vi "获取公式.vi"(10 "量程选择":enum16{"L", "H", "AUTO"}(ring)) -> (2 "方程系数2":cluster{"X^2":dbl, "K":dbl, "b":dbl} {"X^2" format="%#.6g"; "b" format="%#.6g"; "K" format="%#.6g"}, 3 "方程系数":cluster{"X^2":dbl, "K":dbl, "b":dbl} {"X^2" format="%#.6g"; "b" format="%#.6g"; "K" format="%#.6g"})   [LabVIEW 2016, in "斯坦道CODMn.lvlib"]
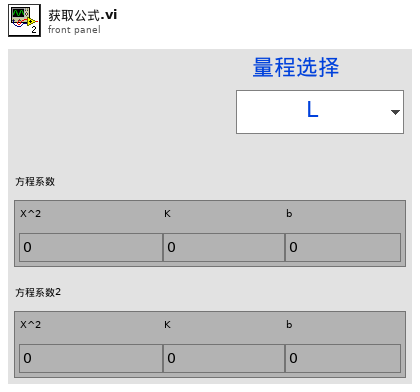
[diagram p1: front panel]
types:
  T1 = cluster{"数组 2[0]":sgl, "数组 2[1]":sgl, "数组 2[2]":sgl, "数组 2[3]":sgl, "数组 2[4]":sgl, "数组 2[5]":sgl, "数组 2[6]":sgl, "数组 2[7]":sgl, "数组 2[8]":sgl, "数组 2[9]":sgl, "数组 2[10]":sgl, "数组 2[11]":sgl, "数组 2[12]":sgl, "数组 2[13]":sgl, "数组 2[14]":sgl, "数组 2[15]":sgl, "数组 2[16]":sgl, "数组 2[17]":sgl, "数组 2[18]":sgl, "数组 2[19]":sgl, "数组 2[20]":sgl, "数组 2[21]":sgl, "数组 2[22]":sgl, "数组 2[23]":sgl, "数组 2[24]":sgl, "数组 2[25]":sgl, "数组 2[26]":sgl, "数组 2[27]":sgl, "数组 2[28]":sgl, "数组 2[29]":sgl, "数组 2[30]":sgl, "数组 2[31]":sgl, "数组 2[32]":sgl, "数组 2[33]":sgl, "数组 2[34]":sgl, "数组 2[35]":sgl, "数组 2[36]":sgl, "数组 2[37]":sgl, "数组 2[38]":sgl, "数组 2[39]":sgl, "数组 2[40]":sgl, "数组 2[41]":sgl}
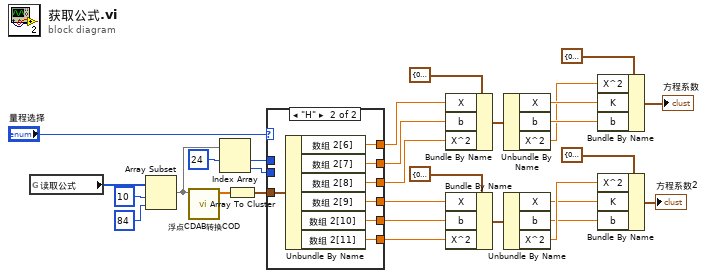
[diagram p0: block diagram]
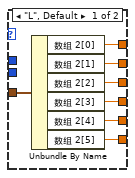
[diagram p2: hidden frame]
diagram:
  n1 = global read "COD内部交互全局.vi" "读取公式"() -> (w30:u16[])
  n2 = Array Subset(array=w30, index=10 ("索引"), length=84 ("长度")) -> (w21:u16[])
  n3 = call "浮点CDAB转换COD.vi"("数组"=w21) -> ("数组 2"=w28:sgl[])  [unwired: 10 in]
  n4 = Index Array(array=w21, index #1=24 ("索引")) -> (element #1=w19:u16, element #2=w18:u16)  [unwired: 1 in]
  n5 = Array To Cluster(array=w28) -> (cluster=w29:T1)
  n6 = case shown="\"H\"" "量程选择" {
    tunnel: w29 -> [w37 w44]
    tunnel: [w36 w43] -> w25
    tunnel: [w35 w42] -> w24
    tunnel: [w34 w41] -> w23
    tunnel: w19 -> [_ _]
    tunnel: w18 -> [_ _]
    tunnel: [w33 w40] -> w16
    tunnel: [w32 w38] -> w15
    tunnel: [w31 w39] -> w14
    frame "L", Default {
      n7 = Unbundle By Name(w37) -> ("数组 2[0]"=w36:sgl, "数组 2[1]"=w35:sgl, "数组 2[2]"=w34:sgl, "数组 2[3]"=w33:sgl, "数组 2[4]"=w32:sgl, "数组 2[5]"=w31:sgl)
    }
    frame "H" {
      n8 = Unbundle By Name(w44) -> ("数组 2[6]"=w43:sgl, "数组 2[7]"=w42:sgl, "数组 2[8]"=w41:sgl, "数组 2[9]"=w40:sgl, "数组 2[10]"=w38:sgl, "数组 2[11]"=w39:sgl)
    }
  }
  n9 = Bundle By Name(cluster=cluster{"X":dbl, "b":dbl, "X^2":dbl} {"X"=0.0, "b"=0.0, "X^2"=0.0} ("方程系数"), "X"=w25, "b"=w24, "X^2"=w23) -> (w12:cluster{"X":dbl, "b":dbl, "X^2":dbl})
  n10 = Bundle By Name(cluster=cluster{"X":dbl, "b":dbl, "X^2":dbl} {"X"=0.0, "b"=0.0, "X^2"=0.0} ("方程系数"), "X"=w16, "b"=w15, "X^2"=w14) -> (w4:cluster{"X":dbl, "b":dbl, "X^2":dbl})
  n11 = Unbundle By Name(w12) -> ("X"=w11:dbl, "b"=w10:dbl, "X^2"=w9:dbl)
  n12 = Unbundle By Name(w4) -> ("X"=w6:dbl, "b"=w7:dbl, "X^2"=w8:dbl)
  n13 = Bundle By Name(cluster=cluster{"X^2":dbl, "K":dbl, "b":dbl} {"X^2"=0.0, "K"=0.0, "b"=0.0} ("方程系数"), "X^2"=w9, "K"=w11, "b"=w10) -> (→"方程系数":cluster{"X^2":dbl, "K":dbl, "b":dbl})
  n14 = Bundle By Name(cluster=cluster{"X^2":dbl, "K":dbl, "b":dbl} {"X^2"=0.0, "K"=0.0, "b"=0.0} ("方程系数"), "X^2"=w8, "K"=w6, "b"=w7) -> (→"方程系数2":cluster{"X^2":dbl, "K":dbl, "b":dbl})
